vi "flow_queue_pickup.vi"(6 "timeout":i32=-1, 8 "error in (no error)":errorcluster caption="エラー入力（エラーなし）", 11 "queue in":refnum<queue>) -> (0 "error out":errorcluster caption="エラー出力", 1 "parameter":variant, 2 "command":string, 3 "queue out":refnum<queue>, 4 "timeout?":bool)   [LabVIEW 2017]
uses:
  flow_queue_datatype.ctl
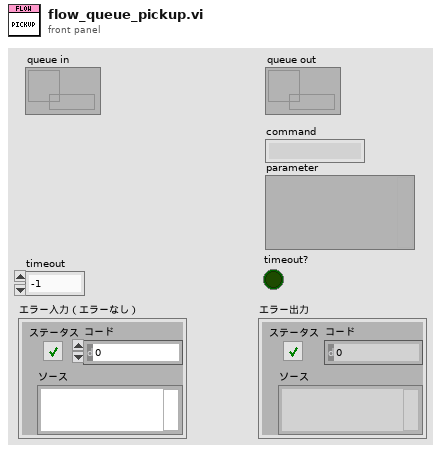
[diagram p1: front panel]
types:
  T1 = typedef "flow_queue_datatype.ctl" = cluster{"command":string, "parameter":variant}
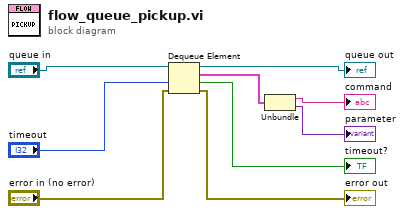
[diagram p0: block diagram]
diagram:
  n1 = Dequeue Element(queue="queue in", timeout in ms (-1)="timeout", error in (no error)="error in (no error)") -> (queue out=→"queue out":refnum<queue>, element=w3:T1, timed out?=→"timeout?":bool, error out=→"error out":errorcluster)
  n2 = Unbundle(w3) -> ("command"=→"command":string, "parameter"=→"parameter":variant)
